vi "ROI entry-Buttons setup.vi"(9 "Acquisition button disabled?":T2(ring), 10 "Done button disabled?":T2(ring), 11 "ROI Enum":T1) -> ()   [LabVIEW 2017]
uses:
  Typedefs/ROI ID Enum.ctl
  ROI Entry screen/Typedefs/ROI input mode.ctl
  ROI Entry screen/Globals/gl_ROI Entry UI globals.vi
panel:
  out "Acq Type":enum16{"Functional Acq", "Volume Acq"}(ring)
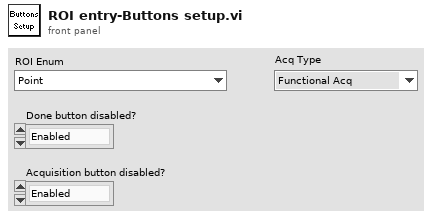
[diagram p1: front panel]
types:
  T1 = typedef "ROI ID Enum.ctl" = enum16{"Point", "MiniScan", "Comp. MiniScan", "Rectangle", "Comp. volume", "Arb. plane point", "None"}
  T2 = enum8{"Enabled", "Disabled", "Disabled and Grayed Out"}
  T3 = typedef "ROI input mode.ctl" = enum16{"Unspecified", "Point-Line-Plane", "Volume"}
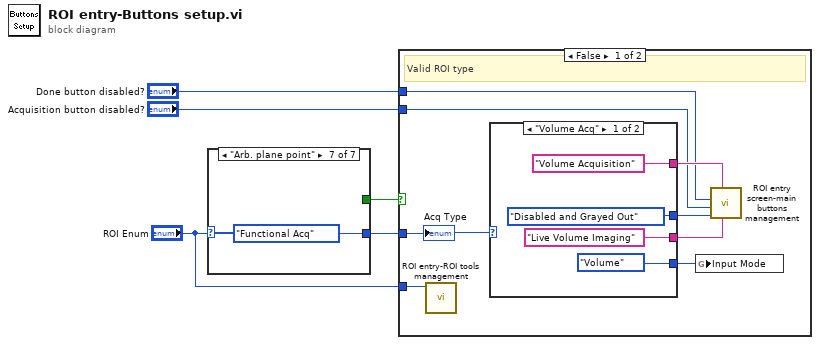
[diagram p0: block diagram]
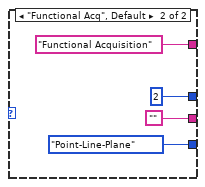
[diagram p2: hidden frame]
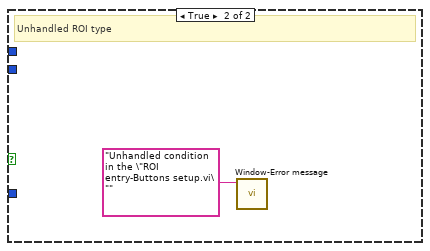
[diagram p3: hidden frame]
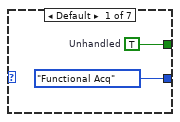
[diagram p4: hidden frame]
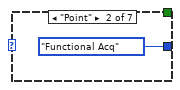
[diagram p5: hidden frame]
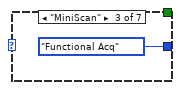
[diagram p6: hidden frame]
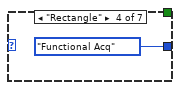
[diagram p7: hidden frame]
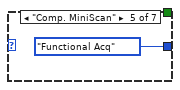
[diagram p8: hidden frame]
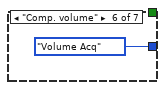
[diagram p9: hidden frame]
diagram:
  n1 = case shown="\"Arb. plane point\"" "ROI Enum" {
    tunnel: [enum16{"Functional Acq", "Volume Acq"}."Functional Acq" ("Acq Type") enum16{"Functional Acq", "Volume Acq"}."Functional Acq" ("Acq Type") enum16{"Functional Acq", "Volume Acq"}."Functional Acq" ("Acq Type") enum16{"Functional Acq", "Volume Acq"}."Functional Acq" ("Acq Type") enum16{"Functional Acq", "Volume Acq"}."Functional Acq" ("Acq Type") enum16{"Functional Acq", "Volume Acq"}."Volume Acq" ("Acq Type") enum16{"Functional Acq", "Volume Acq"}."Functional Acq" ("Acq Type")] -> w3
    tunnel: [w6 _ _ _ _ _ _] -> w2
    frame Default {
      w6 = TRUE  # Unhandled
    }
    frame "Point" {
    }
    frame "MiniScan" {
    }
    frame "Rectangle" {
    }
    frame "Comp. MiniScan" {
    }
    frame "Comp. volume" {
    }
    frame "Arb. plane point" {
    }
  }
  n2 = case shown="False" w2 {
    tunnel: "Done button disabled?" -> [w17 _]
    tunnel: "Acquisition button disabled?" -> [w16 _]
    tunnel: w3 -> [w15 _]
    tunnel: "ROI Enum" -> [w14 _]
    frame False {
      # "Valid ROI type"
      n3 = call "ROI entry-ROI tools management.vi"("ROI Enum"=w14) -> ()  [unwired: 10 in, 1 out]
      n4 = case shown="\"Volume Acq\"" w15 {
        tunnel: [ROI_input_mode."Volume" ("Input Mode") ROI_input_mode."Point-Line-Plane" ("t")] -> w21
        tunnel: [T2."Disabled and Grayed Out" ("Disabled") 2 ("y")] -> w20
        tunnel: ["Volume Acquisition" ("Boolean Text.Text") "Functional Acquisition" ("Boolean Text.Text")] -> w19
        tunnel: ["Live Volume Imaging" ("Boolean Text.Text") "" ("Boolean Text.Text")] -> w18
        frame "Volume Acq" {
        }
        frame "Functional Acq", Default {
        }
      }
      n5 = global write "gl_ROI Entry UI globals.vi" "Input Mode"(w21) -> ()
      n6 = call "ROI entry screen-main buttons management.vi"("Imaging button boolean text"=w18, "Acquisition button boolean text"=w19, "Imaging button disabled?"=w20, "Acquisition button disabled?"=w16, "Done button disabled?"=w17) -> ()  [unwired: 7 in]
      "Acq Type" <- w15
    }
    frame True {
      # "Unhandled ROI type"
      n7 = call "Window-Error message.vi"("Message"="Unhandled condition in the \"ROI entry-Buttons setup.vi\"") -> ()  [unwired: 10 in, 1 out]
    }
  }
